vi "test Main.vi"(8 "error in (no error)":errorcluster, 11 "TestCase in":refnum<class "DBL Pointer Main.lvclass">) -> (0 "error out":errorcluster, 3 "TestCase out":refnum<class "DBL Pointer Main.lvclass">)   [LabVIEW 2017, in "DBL Pointer Main.lvclass"]
uses:
  DBL Pointer Main.lvclass
  Source/Core/Engine/Classes/Pointer/DBL Pointer.lvclass/DBL Pointer.ctl
  <vilib>/NI/Memory Manager/Classes/Pointer/Memory.Pointer.lvclass/Memory.Pointer.ctl
  <vilib>/NI/Memory Manager/Classes/Pointer/Memory.Pointer.Read.vi
  <vilib>/NI/Memory Manager/Classes/Pointer/Memory.Pointer.Read.1D.DBL.vi
  <vilib>/NI/Memory Manager/Classes/Pointer/Memory.Pointer.Parameter Check.Null Pointer.vi
  <vilib>/NI/Memory Manager/Classes/Pointer/Memory.Pointer.Deallocate.vi
  <vilib>/NI/Memory Manager/Classes/Pointer/Memory.Pointer.Read.No Check.1D.DBL.vi
  <vilib>/NI/Memory Manager/Classes/Pointer/Memory.Pointer.Parameter Check.Subset.Power of 2.vi
  <vilib>/NI/Memory Manager/Classes/Pointer/Memory.Pointer.Errors.vi
  <vilib>/NI/Memory Manager/Classes/Pointer/Memory.Pointer.Errors.Null Pointer.vi
  <vilib>/NI/Memory Manager/Classes/Pointer/Memory.Pointer.Get Address.vi
  <vilib>/NI/Memory Manager/Classes/Pointer/Memory.Pointer.Set Address.vi
  <vilib>/NI/Memory Manager/Classes/Pointer/Memory.Pointer.Set Size.vi
  <vilib>/NI/Memory Manager/Classes/Pointer/Memory.Pointer.Set Allocated.vi
  <vilib>/NI/Memory Manager/Classes/Pointer/Memory.Pointer.Errors.Zone.vi
  <vilib>/NI/Memory Manager/Classes/Pointer/Memory.Pointer.Get Allocated.vi
  <vilib>/NI/Memory Manager/Classes/Pointer/Memory.Pointer.Errors.Out of Bounds.vi
  <vilib>/NI/Memory Manager/Classes/Pointer/Memory.Pointer.Get Size.vi
  <vilib>/NI/Memory Manager/Classes/Pointer/Memory.Pointer.Count to Size.Power of 2.vi
  <vilib>/NI/Memory Manager/Classes/Pointer/Memory.Pointer.Errors.Create Error.vi
  <vilib>/NI/Memory Manager/VIs/Source.Write.String.vi
  <vilib>/NI/Memory Manager/Classes/Pointer/Memory.Pointer.Errors.Write Pointer Size.vi
  <vilib>/NI/Memory Manager/VIs/Source.Write.Scalar.Base10.vi
  <vilib>/NI/Memory Manager/VIs/Source.Write.Scalar.Base10 (U64).vi
  <vilib>/NI/Memory Manager/VIs/New Error Cluster Constant.vi
  <vilib>/NI/Memory Manager/VIs/New Error Cluster Constant (512B).vi
  <vilib>/NI/Memory Manager/VIs/Error Cluster.Set Status.vi
  <vilib>/NI/Memory Manager/VIs/Error Cluster.Set Code.vi
  <vilib>/NI/Memory Manager/VIs/Error Cluster.Set VI Source.vi
  <vilib>/NI/Memory Manager/Constants/Memory.Constants.vi
  <vilib>/NI/Memory Manager/Constants/Memory.Constants.Library Name.vi
  <vilib>/NI/Memory Manager/Classes/Pointer/Memory.Pointer.Errors.Get Info.vi
  Source/Core/Engine/Classes/Pointer/DBL Pointer.lvclass
  C:/Program Files (x86)/National Instruments/LabVIEW 2017/vi.lib/NI/Memory Manager/Classes/Pointer/Memory.Pointer.lvclass
  <vilib>/addons/_JKI Toolkits/VI Tester/TestCase.llb/TestCase.lvclass
  <vilib>/NI/Memory Manager/Classes/Pointer/Memory.Pointer.lvclass
  C:/Program Files (x86)/National Instruments/LabVIEW 2017/vi.lib/addons/_JKI Toolkits/VI Tester/TestCase.llb/TestCase.lvclass
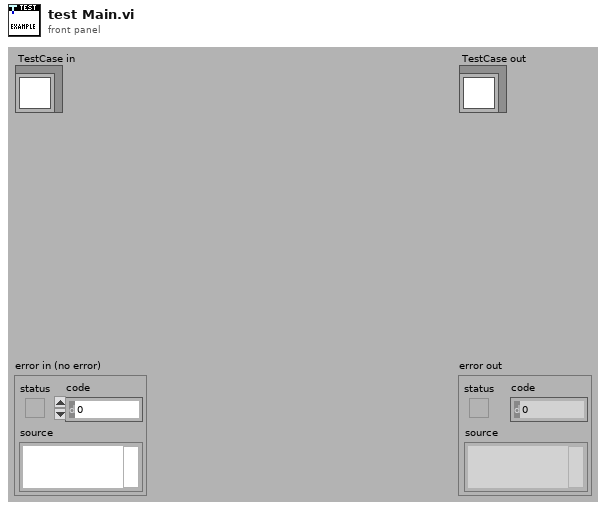
[diagram p1: front panel]
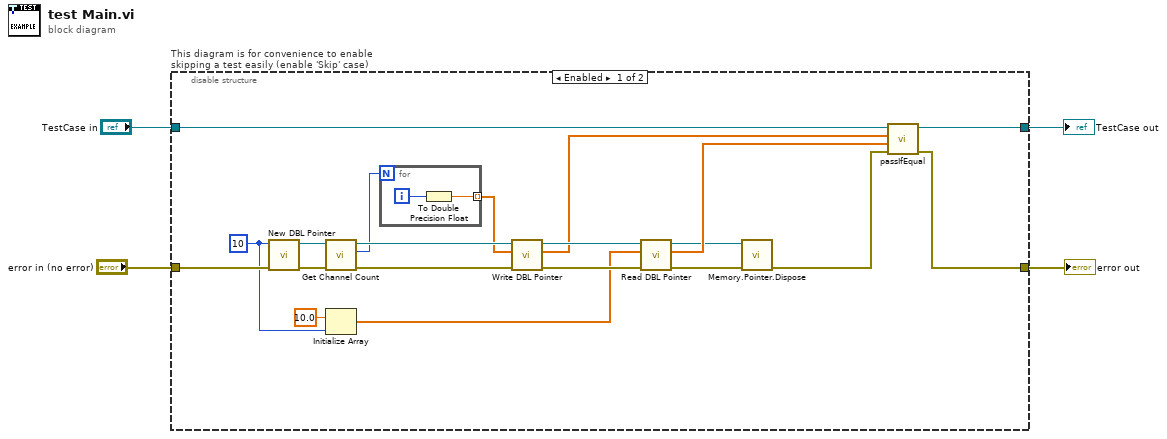
[diagram p0: block diagram]
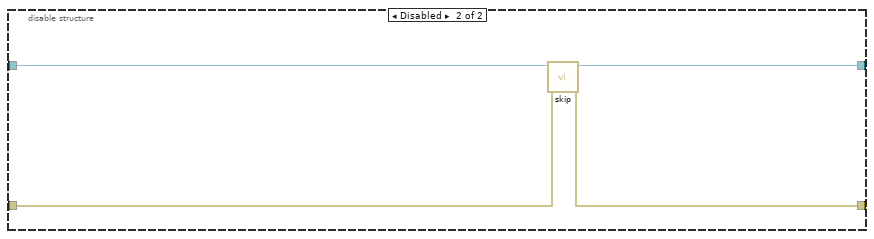
[diagram p2: hidden frame]
diagram:
  n1 = disable-structure "This diagram is for convenience to enable skipping a test easily (enable 'Skip' case)" shown="Enabled" {
    disable-tunnel: "TestCase in" -> [w23 w29]
    disable-tunnel: [w22 w27] -> w1
    disable-tunnel: [w21 w28] -> w3
    disable-tunnel: "error in (no error)" -> [w20 w26]
    frame Enabled {
      w12 = u64 10 ("channel count")
      n2 = call "New DBL Pointer.vi"("error in (no error)"=w20, "channel count"=w12) -> ("error out"=w19:errorcluster, "DBL Pointer out"=w17:refnum<class "DBL Pointer.lvclass">)  [unwired: 8 in]
      n3 = call "Get Channel Count.vi"("DBL Buffer in"=w17) -> ("channel count"=w14:u64, "DBL Buffer out"=w16:refnum<class "DBL Pointer.lvclass">)  [unwired: 9 in]
      n4 = Initialize Array(10.0 ("element"), w12) -> (w10:dbl[])
      n5 = for {
        N: w14 -> [_]
        tunnel: [w24] -> w13 mode=indexing
        i -> [w25]
        n6 = To Double Precision Float(number=w25) -> (double precision float=w24:dbl)
      }
      n7 = call "Write DBL Pointer.vi"("error in (no error)"=w19, "buffer in"=w13, "DBL Pointer in"=w16) -> ("error out"=w18:errorcluster, "buffer out"=w9:dbl[], "DBL Pointer out"=w15:refnum<class "DBL Pointer.lvclass">)  [unwired: 6 in]
      n8 = call "Read DBL Pointer.vi"("error in (no error)"=w18, "buffer in"=w10, "DBL Pointer in"=w15) -> ("error out"=w6:errorcluster, "buffer out"=w8:dbl[], "DBL Pointer out"=w7:refnum<class "DBL Pointer.lvclass">)  [unwired: 6 in]
      n9 = call <vilib>:"Memory.Pointer.Dispose.vi"("error in (no error)"=w6, "Pointer in"=w7) -> ("error out"=w5:errorcluster)  [unwired: 8 in, 1 out]
      n10 = call-dynamic "passIfEqual.vi"("error in (no error)"=w5, "y"=w8, "x"=w9, "TestCase in"=w23) -> ("error out"=w21:errorcluster, "TestCase out"=w22:refnum<class "DBL Pointer Main.lvclass">)  [unwired: 6 in]
    }
    frame Disabled {
      # "skip test result while test is under development"
      n11 = call <vilib>:"skip.vi"("error in (no error)"=w26, "TestCase in"=w29) -> ("error out"=w28:errorcluster, "TestCase out"=w27:refnum<class "DBL Pointer Main.lvclass">)  [unwired: 8 in]
    }
  }
  "error out" <- w3
  "TestCase out" <- w1
